vi "zad2.vi"() -> ()   [LabVIEW 2017]
panel:
  out "Numeric":dbl
  in  "stop":bool
  in  "Knob 3":dbl(knob) scale=0.0..10.0
  in  "Knob 2":dbl(knob) scale=0.0..10.0
  in  "Knob":dbl(knob) scale=0.0..10.0
  out "Waveform Graph":dynamicdata(graph)
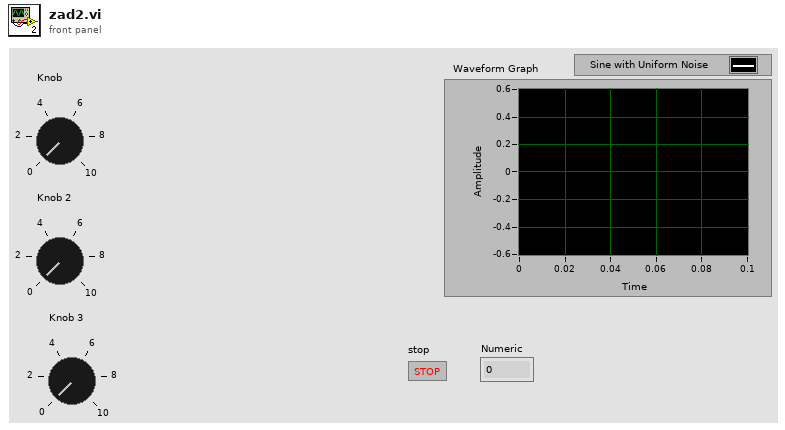
[diagram p1: front panel]
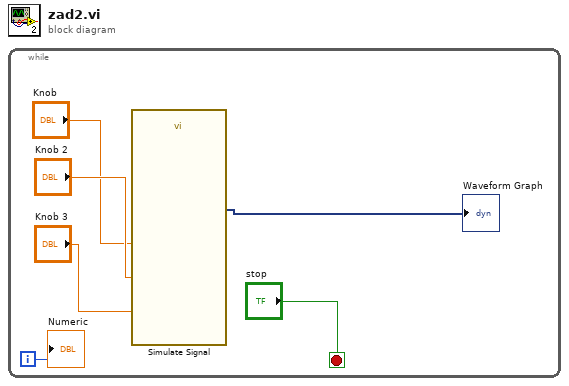
[diagram p0: block diagram]
diagram:
  n1 = while {
    i -> [w5]
    stop <- "stop" stop-if-true
    n2 = call "Simulate Signal"("Offset"="Knob 3", "Frequency"="Knob 2", "Amplitude"="Knob") -> ("Sine with Uniform Noise"=→"Waveform Graph":dynamicdata)  [unwired: 11 in, 1 out]
    "Numeric" <- w5
  }
